vi "MongoDB.CollectionExists.vi"(8 "error in (no error)":errorcluster, 10 "collectionName":string, 11 "MongoDB.Database in":refnum<class "MongoDB.Database.lvclass">) -> (0 "error out":errorcluster, 2 "CollectionExists":bool, 3 "MongoDB.Database out":refnum<class "MongoDB.Database.lvclass">)   [LabVIEW 2014, in "MongoDB.Database.lvclass"]
uses:
  MongoDB.Database.lvclass
  MongoDB.Database.lvclass/MongoDB.Database.ctl
  C:/MongoData/Drivers/mongo-csharp-driver-2.0.0-beta4/mongo-csharp-driver-2.0.0-beta4/src/MongoDB.Driver.Legacy/bin/Release/MongoDB.Driver.Legacy.dll
  MongoData/Drivers/mongo-csharp-driver-2.0.0-beta4/mongo-csharp-driver-2.0.0-beta4/src/MongoDB.Driver.Legacy/bin/Release/MongoDB.Driver.Legacy.dll
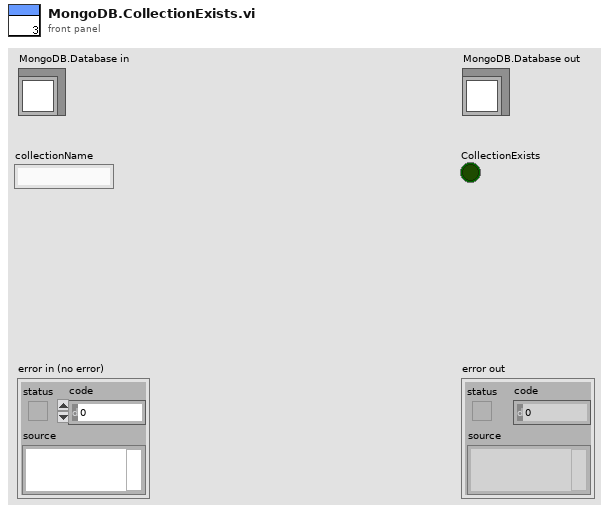
[diagram p1: front panel]
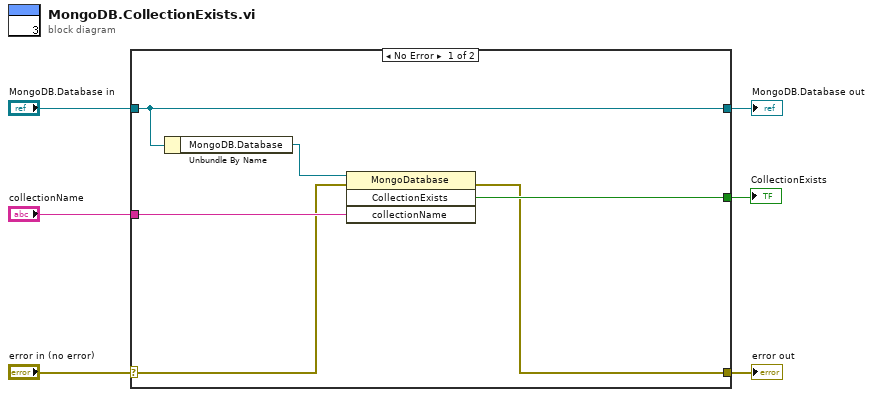
[diagram p0: block diagram]
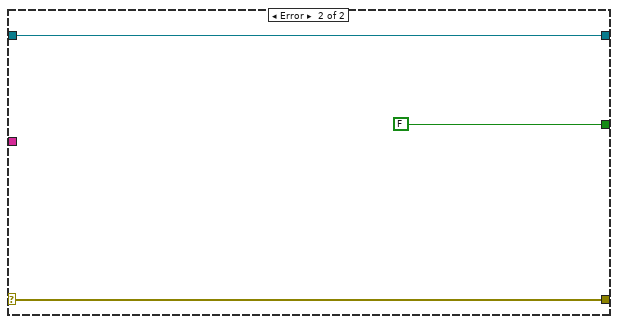
[diagram p2: hidden frame]
diagram:
  n1 = case shown="No Error" "error in (no error)" {
    selector: "error in (no error)" -> [w8 w15]
    tunnel: [w7 w15] -> w5
    tunnel: [w12 w14] -> w3
    tunnel: "MongoDB.Database in" -> [w12 w14]
    tunnel: "collectionName" -> [w10 _]
    tunnel: [w9 FALSE ("CollectionExists")] -> w1
    frame No Error {
      n2 = Unbundle By Name(w12) -> ("MongoDB.Database"=w11:refnum<k24>)
      n3 = invoke class="MongoDatabase" method="CollectionExists"(reference=w11, error in=w8, "collectionName"=w10) -> (error out=w7:errorcluster, "CollectionExists"=w9:bool)  [unwired: 1 in, 2 out]
    }
    frame Error {
    }
  }
  "error out" <- w5
  "MongoDB.Database out" <- w3
  "CollectionExists" <- w1
